vi "Update Display.vi"(8 "error in (no error)":errorcluster, 11 "Products Picker in":refnum<class "Products Picker.lvclass">) -> (0 "error out":errorcluster, 3 "Products Picker out":refnum<class "Products Picker.lvclass">)   [LabVIEW 2020, in "Products Picker.lvlib" / "Products Picker.lvclass"]
uses:
  Products Picker.lvclass
  Products Picker.lvclass/Products Picker.ctl
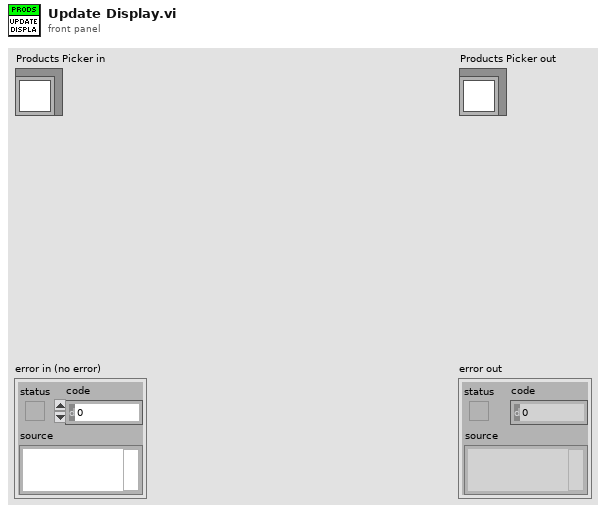
[diagram p1: front panel]
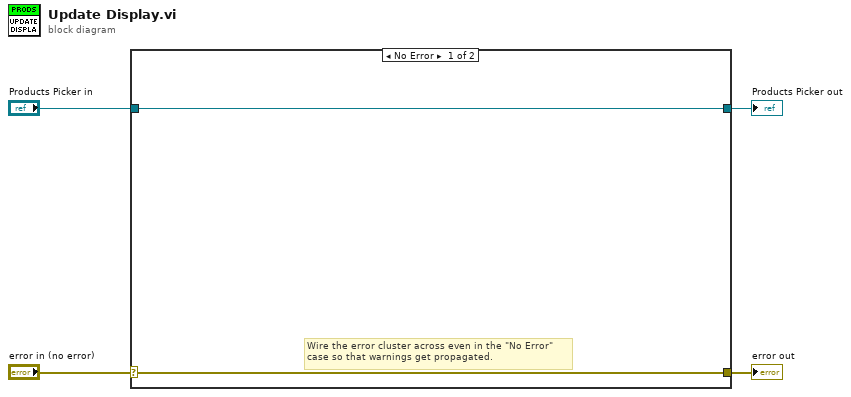
[diagram p0: block diagram]
diagram:
  n1 = case shown="No Error" "error in (no error)" {
    selector: "error in (no error)" -> [w5 w8]
    tunnel: [w5 w8] -> w3
    tunnel: [w6 w7] -> w1
    tunnel: "Products Picker in" -> [w6 w7]
    frame No Error {
      # "Wire the error cluster across even in the \"No Error\"\ncase so that warnings get propagated."
    }
    frame Error {
    }
  }
  "error out" <- w3
  "Products Picker out" <- w1
